vi "lv2012 - VI 2.vi"() -> ()   [LabVIEW 2012]
panel:
  out "String":string
  in  "Stop Button":bool
  out "Event Counter":dbl
  out "Numeric Indicator":dbl
  in  "Enum":enum16{"Init", "Run", "End"}(ring)
  in  "Numeric Control":dbl
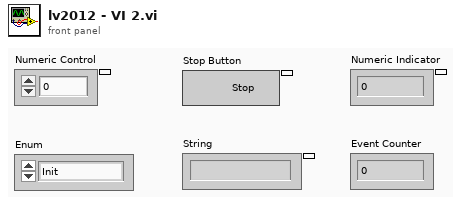
[diagram p1: front panel]
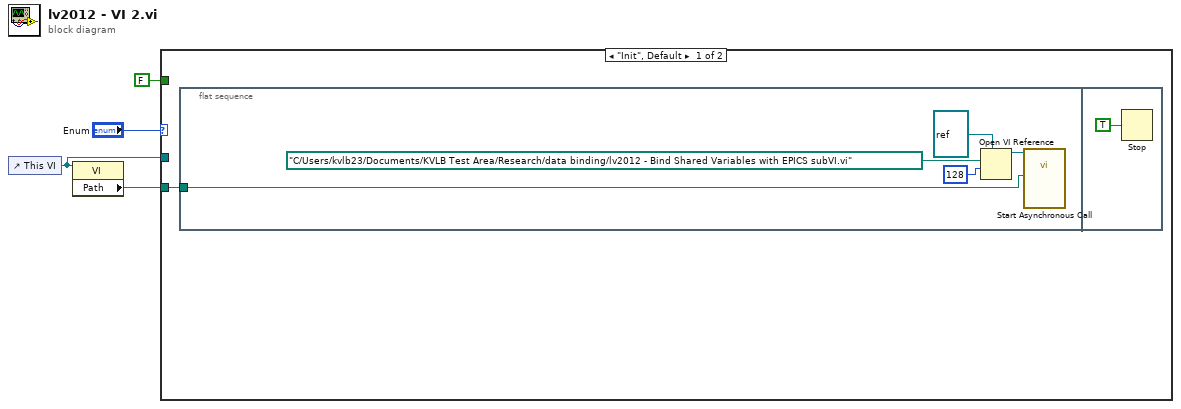
[diagram p0: block diagram]
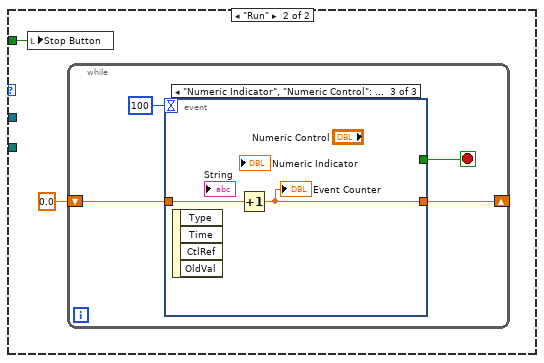
[diagram p2: hidden frame]
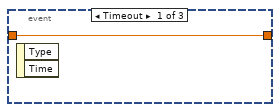
[diagram p3: hidden frame]
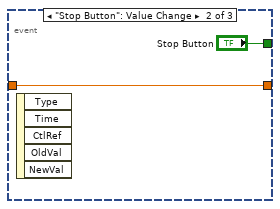
[diagram p4: hidden frame]
diagram:
  n1 = control-ref of="This VI"() -> (w1:refnum<vi>)
  n2 = property class="VI"(reference=w1) -> ("Path"=w2:path)  [unwired: 1 in, 2 out]
  n3 = case shown="\"Init\", Default" "Enum" {
    tunnel: FALSE ("replace all? (F)") -> [_ w12]
    tunnel: w2 -> [w5 _]
    tunnel: w1 -> [_ _]
    frame "Init", Default {
      n4 = flat-sequence {
        tunnel: w5 -> [w6]
        frame #0 {
          n5 = Open VI Reference(type specifier VI Refnum (for type only)=refnum<vi> refnum, vi path=path "C:/Users/kvlb23/Documents/KVLB Test Area/Research/data binding/lv2012 - Bind Shared Variables with EPICS subVI.vi", options=128) -> (vi reference=w7:refnum<vi>)  [unwired: 3 in, 1 out]
          n6 = call-by-ref "Start Asynchronous Call"(reference=w7, "vi path"=w6) -> ()  [unwired: 11 in, 3 out]
        }
        frame #1 {
          n7 = Stop(stop? (T)=TRUE) -> ()
        }
      }
    }
    frame "Run" {
      n8 = local write "Stop Button"(w12) -> ()
      n9 = while {
        shift-right: [w15] -> _
        shift-left: 0.0 -> [w16]
        stop <- w14 stop-if-true
        n10 = event shown="[2] \"Numeric Indicator\", \"Numeric Control\": Value Change" {
          selector: _ -> [_ _ _]
          dyn-events: _ -> [_ _ _]
          timeout: 100 -> [_ _ _]
          tunnel: w16 -> [w18 w20 w22]
          tunnel: [w18 w20 w21] -> w15
          tunnel: [_ "Stop Button" _] -> w14
          event Timeout {
            n11 = event-data() -> ()  [unwired: 1 in, 2 out]
          }
          event "Stop Button": Value Change {
            n12 = event-data() -> ()  [unwired: 1 in, 5 out]
          }
          event "Numeric Indicator", "Numeric Control": Value Change {
            n13 = event-data() -> ()  [unwired: 1 in, 4 out]
            n14 = Increment(x=w22) -> (x+1=w21:dbl)
            "Event Counter" <- w21
          }
        }
      }
    }
  }
